vi "test Loopback.vi"(8 "error in":errorcluster, 11 "TestCase in":refnum<class "Loopback.lvclass">) -> (0 "error out":errorcluster, 3 "TestCase out":refnum<class "Loopback.lvclass">)   [LabVIEW 2020, in "Loopback.lvclass"]
uses:
  Loopback.lvclass
  <vilib>/addons/_JKI Toolkits/VI Tester/TestCase.llb/TestCase.lvclass
  C:/Program Files (x86)/National Instruments/LabVIEW 2020/vi.lib/addons/_JKI Toolkits/VI Tester/TestCase.llb/TestCase.lvclass
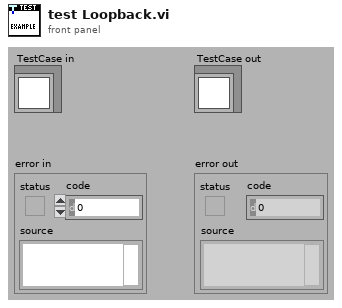
[diagram p1: front panel]
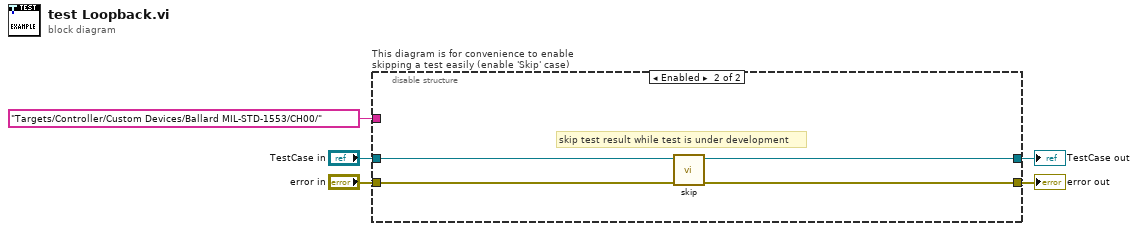
[diagram p0: block diagram]
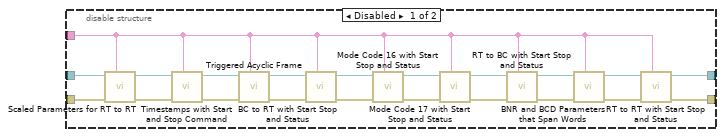
[diagram p2: hidden frame]
diagram:
  n1 = disable-structure "This diagram is for convenience to enable skipping a test easily (enable 'Skip' case)" shown="Enabled" {
    disable-tunnel: "TestCase in" -> [w26 w30]
    disable-tunnel: [w25 w28] -> w2
    disable-tunnel: [w24 w29] -> w4
    disable-tunnel: "error in" -> [w23 w27]
    disable-tunnel: "Targets/Controller/Custom Devices/Ballard MIL-STD-1553/CH00/" ("Channel") -> [w22 _]
    frame Disabled {
      n2 = call "Scaled Parameters for RT to RT.vi"("base name for channel aliases"=w22, "error in"=w23, "Loopback in"=w26) -> ("error out"=w20:errorcluster, "Loopback out"=w21:refnum<class "Loopback.lvclass">)  [unwired: 7 in]
      n3 = call "Timestamps with Start and Stop Command.vi"("base name for channel aliases"=w22, "error in"=w20, "Loopback in"=w21) -> ("error out"=w18:errorcluster, "Loopback out"=w19:refnum<class "Loopback.lvclass">)  [unwired: 7 in]
      n4 = call "Triggered Acyclic Frame.vi"("base name for channel aliases"=w22, "error in"=w18, "Loopback in"=w19) -> ("error out"=w16:errorcluster, "Loopback out"=w17:refnum<class "Loopback.lvclass">)  [unwired: 7 in]
      n5 = call "BC to RT with Start Stop and Status.vi"("base name for channel aliases"=w22, "error in"=w16, "Loopback in"=w17) -> ("error out"=w14:errorcluster, "Loopback out"=w15:refnum<class "Loopback.lvclass">)  [unwired: 7 in]
      n6 = call "Mode Code 16 with Start Stop and Status.vi"("base name for channel aliases"=w22, "error in"=w14, "Loopback in"=w15) -> ("error out"=w12:errorcluster, "Loopback out"=w13:refnum<class "Loopback.lvclass">)  [unwired: 7 in]
      n7 = call "Mode Code 17 with Start Stop and Status.vi"("base name for channel aliases"=w22, "error in"=w12, "Loopback in"=w13) -> ("error out"=w10:errorcluster, "Loopback out"=w11:refnum<class "Loopback.lvclass">)  [unwired: 7 in]
      n8 = call "RT to BC with Start Stop and Status.vi"("base name for channel aliases"=w22, "error in"=w10, "Loopback in"=w11) -> ("error out"=w8:errorcluster, "Loopback out"=w9:refnum<class "Loopback.lvclass">)  [unwired: 7 in]
      n9 = call "BNR and BCD Parameters that Span Words.vi"("base name for channel aliases"=w22, "error in"=w8, "Loopback in"=w9) -> ("error out"=w6:errorcluster, "Loopback out"=w7:refnum<class "Loopback.lvclass">)  [unwired: 7 in]
      n10 = call "RT to RT with Start Stop and Status.vi"("base name for channel aliases"=w22, "error in"=w6, "Loopback in"=w7) -> ("error out"=w24:errorcluster, "Loopback out"=w25:refnum<class "Loopback.lvclass">)  [unwired: 7 in]
    }
    frame Enabled {
      # "skip test result while test is under development"
      n11 = call <vilib>:"skip.vi"("error in (no error)"=w27, "TestCase in"=w30) -> ("error out"=w29:errorcluster, "TestCase out"=w28:refnum<class "Loopback.lvclass">)  [unwired: 8 in]
    }
  }
  "error out" <- w4
  "TestCase out" <- w2
